vi "String NotContain.vi"(11 "Data In":string) -> (3 "Data Out":string)   [LabVIEW 2016]
uses:
  Core/Assert API Components/Failure Actions.ctl
  Core/Assert API Components/Assert API Components.lvlib
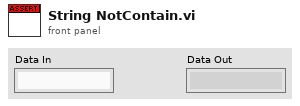
[diagram p1: front panel]
types:
  T1 = typedef "Assert API Components.lvlib/Failure Actions.ctl" = enum16{"None", "Log To File", "Pause Execution", "Abort Execution"}
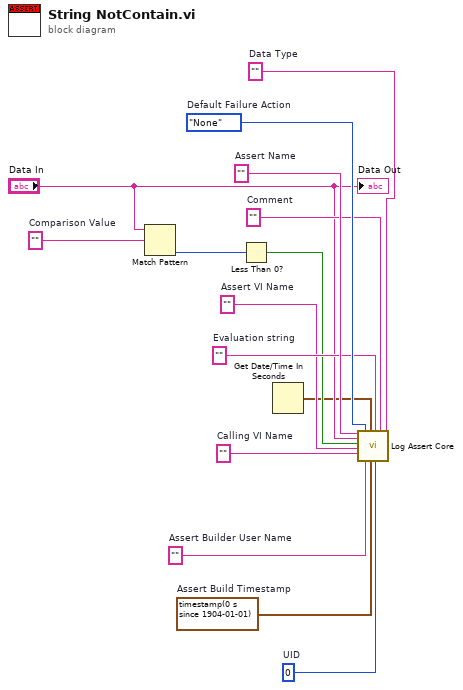
[diagram p0: block diagram]
diagram:
  w1 = 0  # UID
  w3 = ""  # Assert VI Name
  w4 = ""  # Calling VI Name
  w5 = ""  # Assert Builder User Name
  w6 = timestamp(0 s since 1904-01-01)  # Assert Build Timestamp
  w7 = ""  # Data Type
  w13 = ""  # Comment
  w12 = ""  # Evaluation string
  w14 = Failure_Actions."None"  # Default Failure Action
  w15 = ""  # Assert Name
  w10 = ""  # Comparison Value
  n1 = Match Pattern(string="Data In", regular expression=w10) -> (offset past match=w9:i32)  [unwired: 1 in, 3 out]
  n2 = Less Than 0?(x=w9) -> (x < 0?=w8:bool)
  n3 = Get Date/Time In Seconds() -> (seconds since 1Jan1904=w2:timestamp)
  n4 = call "Log Assert Core.vi"("Assert Name"=w15, "Data Value"="Data In", "Status"=w8, "Assert VI Name"=w3, "Calling VI Name"=w4, "Failure Action"=w14, "Assert Builder User Name"=w5, "Last Update"=w2, "Assert Build Timestamp"=w6, "Evaluation String"=w12, "Assert VI UID"=w1, "Comment"=w13, "Data Type"=w7) -> ()  [unwired: 7 in]
  "Data Out" <- "Data In"
